vi "AI Configure Trigger.vi"(8 "error in (no error)":errorcluster, 10 "Params":variant, 11 "Analog Input in":refnum<class "Analog Input.lvclass">) -> (0 "error out":errorcluster, 3 "Analog Input out":refnum<class "Analog Input.lvclass">)   [LabVIEW 2020, in "Instrument.lvlib" / "Analog Input.lvclass"]
uses:
  Analog Input.lvclass
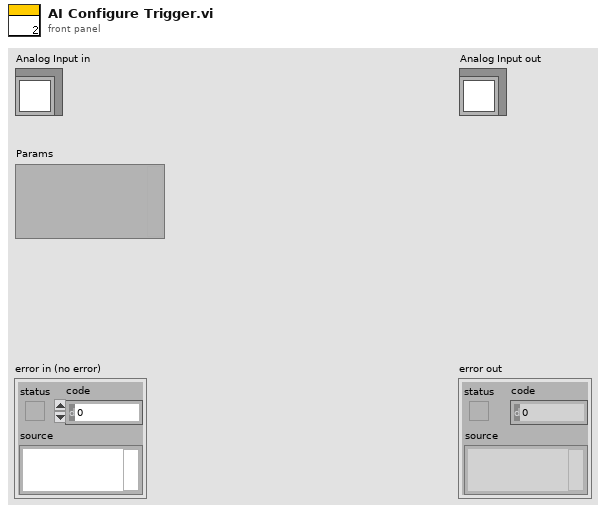
[diagram p1: front panel]
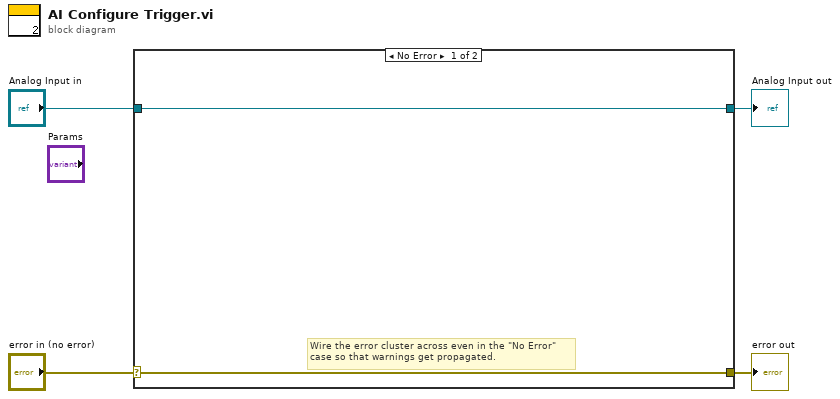
[diagram p0: block diagram]
diagram:
  n1 = case shown="No Error" "error in (no error)" {
    selector: "error in (no error)" -> [w5 w8]
    tunnel: [w5 w8] -> w3
    tunnel: [w6 w7] -> w1
    tunnel: "Analog Input in" -> [w6 w7]
    frame No Error {
      # "Wire the error cluster across even in the \"No Error\"\ncase so that warnings get propagated."
    }
    frame Error {
    }
  }
  "error out" <- w3
  "Analog Input out" <- w1
